vi "parseBoardData.vi"(11 "Array in":string[](array[string])) -> (3 "Array out":i32[][][](array[numeric]))   [LabVIEW 2017]
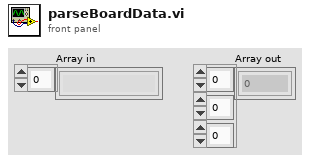
[diagram p1: front panel]
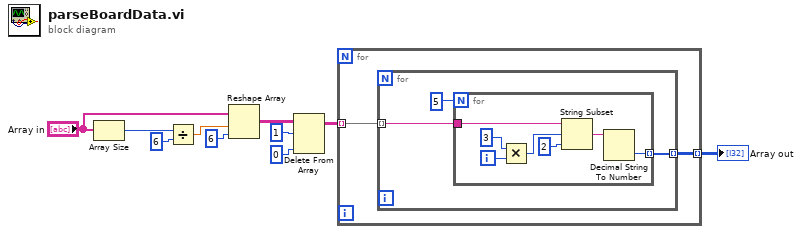
[diagram p0: block diagram]
diagram:
  n1 = Array Size(array="Array in") -> (size(s)=w3:i32)
  n2 = Divide(x=w3, y=6) -> (x/y=w5:dbl)
  n3 = Reshape Array("Array in", w5, 6 ("dimension size")) -> (w6:string[][])
  n4 = Delete From Array(array=w6, length=1, index (col)=0 ("disabled index (col)")) -> (array with subset deleted=w9:string[][])  [unwired: 1 in, 1 out]
  n5 = for {
    tunnel: w9 -> [w12] mode=indexing
    tunnel: [w11] -> w10 mode=indexing
    n6 = for {
      tunnel: w12 -> [w15] mode=indexing
      tunnel: [w13] -> w11 mode=indexing
      n7 = for {
        N: 5 -> [_]
        tunnel: w15 -> [w22]
        tunnel: [w16] -> w13 mode=indexing
        i -> [w21]
        n8 = Multiply(x=3, y=w21) -> (x*y=w19:i32)
        n9 = String Subset(string=w22, offset (0)=w19, length (rest)=2 ("length (rest)")) -> (substring=w17:string)
        n10 = Decimal String To Number(string=w17) -> (number=w16:i32)  [unwired: 2 in, 1 out]
      }
    }
  }
  "Array out" <- w10
